vi "Set Toggle Bit.vi"(10 "Toggle Bit":bool, 11 "Service Data Object in":refnum<class "Service Data Object.lvclass">) -> (3 "Service Data Object out":refnum<class "Service Data Object.lvclass">)   [LabVIEW 2024, in "Service Data Object.lvclass"]
uses:
  Service Data Object.lvclass
  Service Data Object.lvclass/Service Data Object.ctl
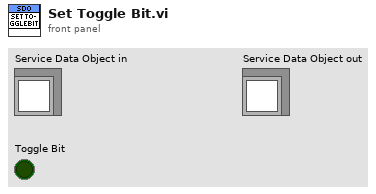
[diagram p1: front panel]
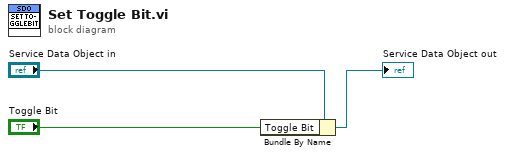
[diagram p0: block diagram]
diagram:
  n1 = Bundle By Name(cluster="Service Data Object in", "Toggle Bit"="Toggle Bit") -> (→"Service Data Object out":refnum<class "Service Data Object.lvclass">)
